vi "ExTestInfoGlbMult.vi"() -> ()   [LabVIEW 2010]
uses:
  GlbCamHndls.vi
panel:
  out "Current Turret":u32
  out "Current Grating":u32
  out "Current Speed":dbl format="%.2f"
  out "Current Wavelength":dbl format="%.2f"
  out "serial number":string
  out "Model number":string
  out "Model number":u32
  in  "Spectrometer number":u32=1 min=1 step=1
  out "error out":errorcluster
  in  "error in (no error)":errorcluster
  # "ExTestInfoGlbMult.vi : this vi reads information from \nspectrometers. It uses gloable varialbes for the \nspectrometer handle. So the spectrometers must \nbe opened before running the program.\nOnce opened this vi can be called any number of times."
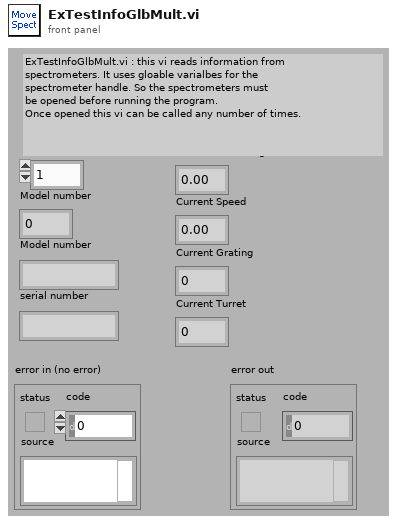
[diagram p1: front panel]
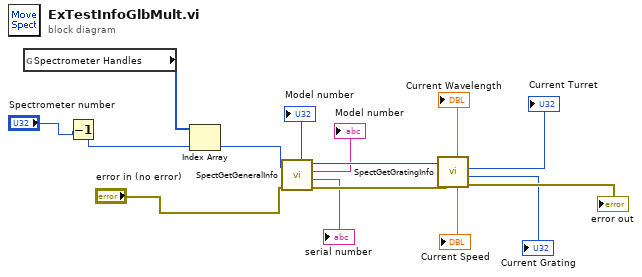
[diagram p0: block diagram]
diagram:
  n1 = global read "GlbCamHndls.vi" "Spectrometer Handles"() -> (w13:u32[])
  n2 = Decrement(x="Spectrometer number") -> (x-1=w14:u32)
  n3 = Index Array(array=w13, index=w14) -> (element=w12:u32)
  n4 = call <userlib>:"SpectGetGeneralInfo.vi"("error in"="error in (no error)", "Spectrometer Handle"=w12) -> ("error out"=w10:errorcluster, "Serial Number"=→"serial number":string, "ModelName"=→"Model number":string, "Spectrometer Handle"=w8:u32, "Model Number"=→"Model number":u32)
  n5 = call <userlib>:"SpectGetGratingInfo.vi"("Spectrometer Handle"=w8, "error in"=w10) -> ("Current Wavelength"=→"Current Wavelength":dbl, "Current Speed"=→"Current Speed":dbl, "Current Turret"=→"Current Turret":i16, "Current Grating"=→"Current Grating":i16, "error out"=→"error out":errorcluster)  [unwired: 1 out]
